vi "Initialize-object.vi"(8 "error in (no error)":errorcluster, 10 "Settings":T1) -> (0 "error out":errorcluster, 3 "Reference out":T3)   [LabVIEW 2013, in "SLMServer.lvlib" / "SLMServer.lvclass"]
uses:
  SLMServer.lvclass
  Object-reference.ctl
  Settings.ctl
  Supported-module-types.ctl
  SLMServer.lvclass/SLMServer.ctl
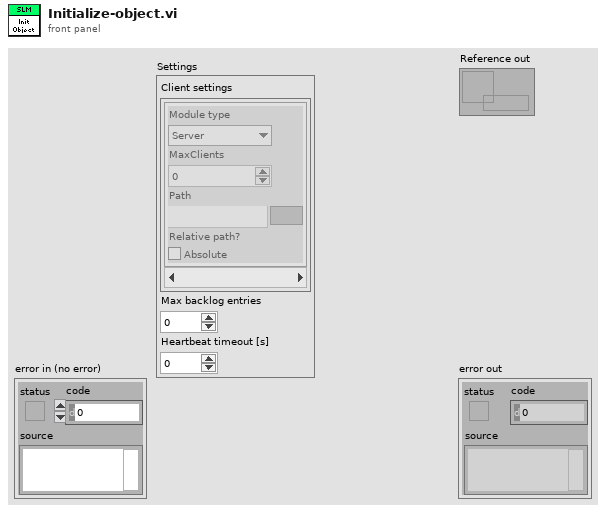
[diagram p1: front panel]
types:
  T1 = typedef "SLMServer.lvlib/SLMServer.lvclass/Settings.ctl" = cluster{"Client settings":cluster{"Module type":T2, "MaxClients":i32, "Path":path, "Relative path?":bool}[], "Max backlog entries":i32, "Heartbeat timeout":dbl}
  T2 = typedef "SLMServer.lvlib/SLMServer.lvclass/Supported-module-types.ctl" = enum16{"SLMControl", "PowderDeposition", "CameraVision", "Server", "All", "StrategyParser", "MaterialCharacterization", "StatusMonitor", "SLMSimulation", "LaserCharacterization"}
  T3 = typedef "SLMServer.lvlib/SLMServer.lvclass/Object-reference.ctl" = refnum<data-value>
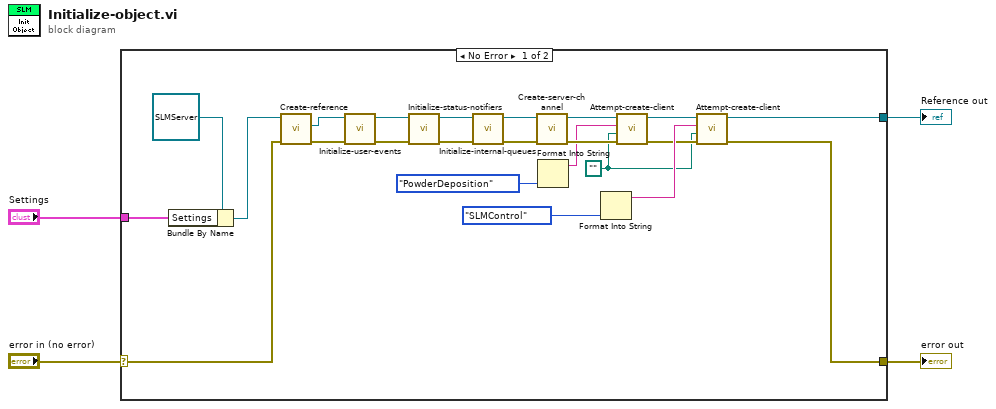
[diagram p0: block diagram]
diagram:
  n1 = case shown="No Error" "error in (no error)" {
    selector: "error in (no error)" -> [w27 w28]
    tunnel: [w7 w28] -> w3
    tunnel: [w6 _] -> w2
    tunnel: "Settings" -> [w24 _]
    frame No Error {
      w5 = path ""
      n2 = Bundle By Name(cluster=refnum<class "SLMServer.lvclass"> refnum ("Panes.lvclass"), "Settings"=w24) -> (w25:refnum<class "SLMServer.lvclass">)
      n3 = call "Create-reference.vi"("error in (no error)"=w27, "Object in"=w25) -> ("error out"=w22:errorcluster, "Object reference"=w23:T3)  [unwired: 7 in, 1 out]
      n4 = call "Initialize-user-events.vi"("error in (no error)"=w22, "ModComm in"=w23) -> ("error out"=w20:errorcluster, "ModComm out"=w21:T3)  [unwired: 8 in]
      n5 = call "Initialize-status-notifiers.vi"("error in (no error)"=w20, "ModComm in"=w21) -> ("error out"=w18:errorcluster, "ModComm out"=w19:T3)  [unwired: 8 in]
      n6 = call "Initialize-internal-queues.vi"("error in (no error)"=w18, "ModComm in"=w19) -> ("error out"=w16:errorcluster, "ModComm out"=w17:T3)  [unwired: 8 in]
      n7 = call "Create-server-channel.vi"("error in (no error)"=w16, "ModComm in"=w17) -> ("error out"=w14:errorcluster, "ModComm out"=w15:T3)  [unwired: 7 in, 1 out]
      n8 = Format Into String(Supported-module-types."PowderDeposition" ("Module type")) -> (resulting string=w12:string)  [unwired: 3 in, 1 out]
      n9 = Format Into String(Supported-module-types."SLMControl" ("Module type")) -> (resulting string=w9:string)  [unwired: 3 in, 1 out]
      n10 = call "Attempt-create-client.vi"("error in (no error)"=w14, "Module path"=w5, "Module type"=w12, "ModComm in"=w15) -> ("error out"=w8:errorcluster, "ModComm out"=w11:T3)  [unwired: 6 in]
      n11 = call "Attempt-create-client.vi"("error in (no error)"=w8, "Module path"=w5, "Module type"=w9, "ModComm in"=w11) -> ("error out"=w7:errorcluster, "ModComm out"=w6:T3)  [unwired: 6 in]
    }
    frame Error {
    }
  }
  "error out" <- w3
  "Reference out" <- w2
